vi "flt_sos4xblock.vi"(7 "sosBypass":bool[](array[boolean])=[FALSE, FALSE, FALSE, FALSE], 8 "input valid":bool, 9 "b":fxp<+/-,24,8>[](array[numeric])=[0.0, 0.0, 0.0, 0.0, 0.0, 0.0, 0.0, 0.0, 0.0, 0.0, 0.0, 0.0], 10 "anot":fxp<+/-,24,8>[](array[numeric])=[0.0, 0.0, 0.0, 0.0, 0.0, 0.0, 0.0, 0.0], 11 "input":fxp<+/-,28,1>) -> (0 "ready for input":bool, 1 "output valid":bool, 3 "output":fxp<+/-,20,2>)   [LabVIEW 2016]
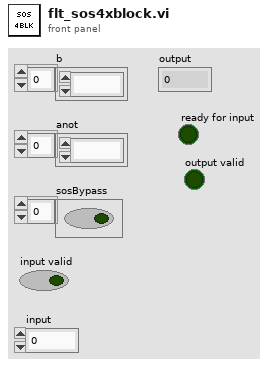
[diagram p1: front panel]
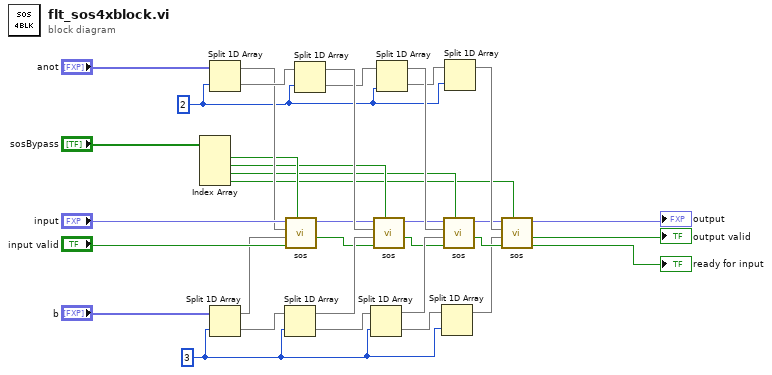
[diagram p0: block diagram]
diagram:
  w8 = 3 ("length")
  w12 = 2 ("length")
  n1 = Index Array(array="sosBypass") -> (element #1=w6:bool, element #2=w5:bool, element #3=w4:bool, element #4=w3:bool)  [unwired: 4 in]
  n2 = Split 1D Array(array="anot", index=w12) -> (first subarray=w22:fxp<+/-,24,8>[], second subarray=w23:fxp<+/-,24,8>[])
  n3 = Split 1D Array(array="b", index=w8) -> (first subarray=w31:fxp<+/-,24,8>[], second subarray=w28:fxp<+/-,24,8>[])
  n4 = Split 1D Array(array=w28, index=w8) -> (first subarray=w30:fxp<+/-,24,8>[], second subarray=w29:fxp<+/-,24,8>[])
  n5 = call "sos.vi"("bypass"=w6, "input valid"="input valid", "b"=w31, "anot"=w22, "input"="input") -> ("output valid"=w20:bool, "output"=w18:fxp<+/-,26,9>)  [unwired: 4 in, 1 out]
  n6 = Split 1D Array(array=w23, index=w12) -> (first subarray=w25:fxp<+/-,24,8>[], second subarray=w24:fxp<+/-,24,8>[])
  n7 = Split 1D Array(array=w29, index=w8) -> (first subarray=w34:fxp<+/-,24,8>[], second subarray=w10:fxp<+/-,24,8>[])
  n8 = call "sos.vi"("bypass"=w5, "input valid"=w20, "b"=w30, "anot"=w25, "input"=w18) -> ("output valid"=w19:bool, "output"=w17:fxp<+/-,26,9>)  [unwired: 4 in, 1 out]
  n9 = Split 1D Array(array=w24, index=w12) -> (first subarray=w26:fxp<+/-,24,8>[], second subarray=w13:fxp<+/-,24,8>[])
  n10 = Split 1D Array(array=w10, index=w8) -> (first subarray=w9:fxp<+/-,24,8>[])  [unwired: 1 out]
  n11 = call "sos.vi"("bypass"=w4, "input valid"=w19, "b"=w34, "anot"=w26, "input"=w17) -> ("output valid"=w16:bool, "output"=w2:fxp<+/-,26,9>)  [unwired: 4 in, 1 out]
  n12 = Split 1D Array(array=w13, index=w12) -> (first subarray=w11:fxp<+/-,24,8>[])  [unwired: 1 out]
  n13 = call "sos.vi"("bypass"=w3, "input valid"=w16, "b"=w9, "anot"=w11, "input"=w2) -> ("ready for input"=→"ready for input":bool, "output valid"=→"output valid":bool, "output"=→"output":fxp<+/-,26,9>)  [unwired: 4 in]
